vi "GOOP_CheckForNewRelease.vi"(10 "QueueRef":refnum<queue>) -> ()   [LabVIEW 2020]
uses:
  <vilib>/httpClient/LabVIEWHTTPClient.lvlib
panel:
  out "Versions":T1
  out "error out":errorcluster
  # "OpenGDS_[\\2E0-9]+[~_]+_LV%s-%s.zip"
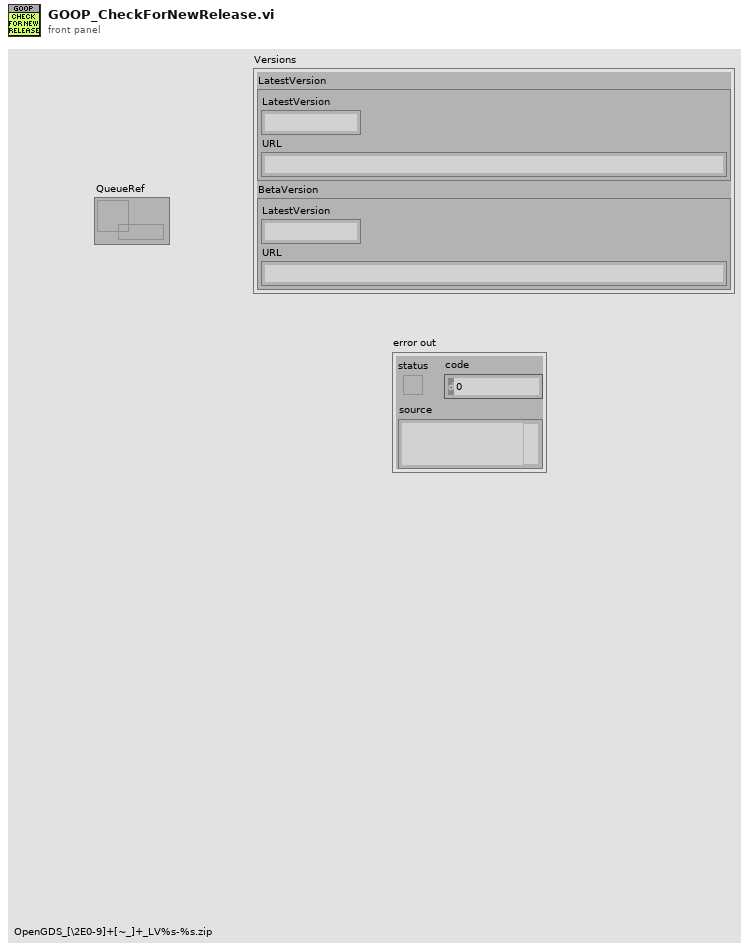
[diagram p1: front panel]
types:
  T1 = cluster{"LatestVersion":cluster{"LatestVersion":string, "URL":string}, "BetaVersion":cluster{"LatestVersion":string, "URL":string}}
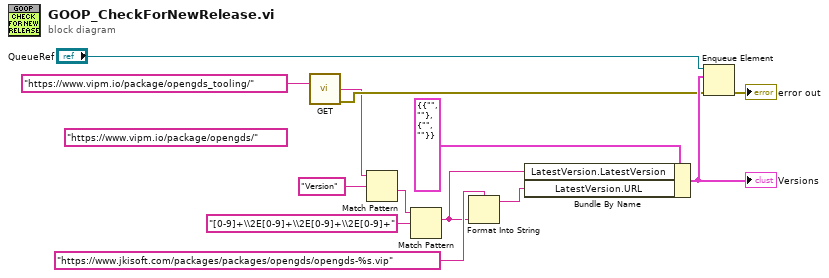
[diagram p0: block diagram]
diagram:
  (unwired) "https://www.vipm.io/package/opengds/" ("url")
  n1 = call <vilib>:"GET.vi"("url"="https://www.vipm.io/package/opengds_tooling/") -> ("body"=w7:string, "error out"=w10:errorcluster)  [unwired: 11 in, 2 out]
  n2 = Match Pattern(string=w7, regular expression="Version") -> (after substring=w5:string)  [unwired: 1 in, 3 out]
  n3 = Match Pattern(string=w5, regular expression="[0-9]+\\2E[0-9]+\\2E[0-9]+\\2E[0-9]+") -> (match substring=w3:string)  [unwired: 1 in, 3 out]
  n4 = Format Into String(format string="https://www.jkisoft.com/packages/packages/opengds/opengds-%s.vip" ("url"), w3) -> (resulting string=w2:string)  [unwired: 2 in, 1 out]
  n5 = Bundle By Name(cluster=T1 {"LatestVersion"={"LatestVersion"="", "URL"=""}, "BetaVersion"={"LatestVersion"="", "URL"=""}} ("output cluster"), "LatestVersion.LatestVersion"=w3, "LatestVersion.URL"=w2) -> (w12:T1)
  "Versions" <- w12
  n6 = Enqueue Element(queue="QueueRef", element=w12, error in (no error)=w10) -> (error out=→"error out":errorcluster)  [unwired: 1 in, 2 out]
